vi "FPGA VI_8 Channels.vi"() -> ()   [LabVIEW 2015]
uses:
  FPGA/Injection Capture IP/Types/Injection.Timing.ctl
  FPGA/Injection Capture IP/Types/Injection.Core.Settings.ctl
  FPGA/Injection Capture IP/Types/Injection.Global.Settings.ctl
  FPGA/Injection Capture IP/Types/Injection.Mux.State.ctl
  <vilib>/Platform/TimedLoop/XDataNode/timing_clust.ctl
  <vilib>/Platform/TimedLoop/XDataNode/nitl_modes.ctl
  <vilib>/Platform/TimedLoop/XDataNode/wakeup.ctl
  FPGA/Injection Capture IP/Types/Injection.Core.Internal.Settings.ctl
  <vilib>/rvi/Emulation/niFpgaGetClockAttributes.vi
  <vilib>/rvi/Emulation/niFpgaSctlEmulationGetInTimedLoop.vi
  <vilib>/rvi/Emulation/niFpgaEmulationReportErrorSimple.vi
  <vilib>/rvi/eio/common/nirviEmuTemplateMethod_errors.vi
  <vilib>/rvi/Emulation/niFpgaCriticalErrorInLSC.vi
  <vilib>/rvi/DataTransferAndStorage/Container/Common/niFpgaContainerExecOnDevCompGetState.vi
  <vilib>/rvi/Emulation/niFpgaEmulationIsFPGAContextNoSignature.vi
  <vilib>/rvi/errors/niFpgaSetErrorForExecOnDevCompSimple.vi
  <vilib>/rvi/eio/common/nirviEmuReportErrorAndStop.vi
  <vilib>/rvi/DataTransferAndStorage/Container/Common/niFpgaContainerGetUniqueNameForEmu.vi
  <vilib>/rvi/FIFO/Fifo_Resource/nirvififoEmulationSetSize.vi
  <vilib>/rvi/FIFO/Fifo_Resource/nirviFifoEmulationQueueMgr.vi
  <instcachedir>/0/nirviFifoEmulationQueueMgr_E5CAEC123FF24DC58D834DCA3CDAA9B5.lvgen/nirviFifoEmulationQueueMgr_E5CAEC123FF24DC58D834DCA3CDAA9B5_010.vi
  <vilib>/rvi/FIFO/Fifo_Resource/nirvififoEmulationDetermineInputValidOut.vi
  <vilib>/rvi/FIFO/Fifo_Resource/nirvififoEmulationCreateLock.vi
  <vilib>/rvi/Emulation/niFpgaProcessEmulError.vi
  <vilib>/rvi/FIFO/Fifo_Resource/nirvififoEmulationObtainLock.vi
  <vilib>/rvi/FIFO/Fifo_Resource/nirvififoEmulationReleaseLock.vi
  <vilib>/rvi/occurrence/nirviWaitOnOccurrenceBase.vi
  <vilib>/rvi/errors/nirviReportUnexpectedCaseInternalError.vi
  <vilib>/rvi/errors/nirviReportUnexpectedCaseInternalError (U32).vi
  <vilib>/Utility/error.llb/Clear Errors.vi
  <vilib>/rvi/interface/RandomDataEmulation/niFpgaRandomDataHandleErrors.vi
  <instcachedir>/0/nirviFifoEmulationQueueMgr_E5CAEC123FF24DC58D834DCA3CDAA9B5.lvgen/nirviFifoEmulationQueueMgr_E5CAEC123FF24DC58D834DCA3CDAA9B5_008.vi
  <vilib>/eio/EIONode/EIONode.xnode
  <vilib>/Platform/TimedLoop/XDataNode/XDataNode.xnode
  <vilib>/rvi/DataTransferAndStorage/Container/XNode/niFpgaContainer.xnode
  <vilib>/rvi/FIFO/Fifo_Resource/niFpgaFifoEmulationRefIn.vi
  <vilib>/rvi/interface/RandomDataEmulation/nirviRandomDataFpgaReadWriteTemplate.vi
  <vilib>/Platform/TimedLoop/XDataNode/XDNodeRunTimeDep.lvlib
panel:
  in  "Settings.DMA":cluster{"# of Injectors":u8}={"# of Injectors"=6}
  out "Host DMA Out?":bool
  out "Intermediate Time Out?":bool
  in  "Settings.Index6.Injectors.Injector6":T1
  in  "Settings.Index7.Injectors.Injector7":T1
  out "Intermediate FIFO Write Timeout":bool
  in  "Settings.Global.Injectors":T2={"Enable?"=FALSE, "Initial Voltage Threshold"=12.0, "Event Dwell Limit"=2000, "Voltage Gain"=1.0, "Current Gain"=1.0, "Filter Samples"=5, "Pretrigger Samples"=5, "Active Edge"=TRUE}
  in  "Settings.Index0.Injectors.Injector0":T1
  in  "Settings.Index1.Injectors.Injector1":T1
  in  "Settings.Index2.Injectors.Injector2":T1
  in  "Settings.Index3.Injectors.Injector3":T1
  in  "Settings.Index4.Injectors.Injector4":T1
  in  "Settings.Index5.Injectors.Injector5":T1
  in  "Settings.Timing":T3={"Injection Sample Period (Ticks)"=80}
  out "Acqusition Loop Ticks":u32
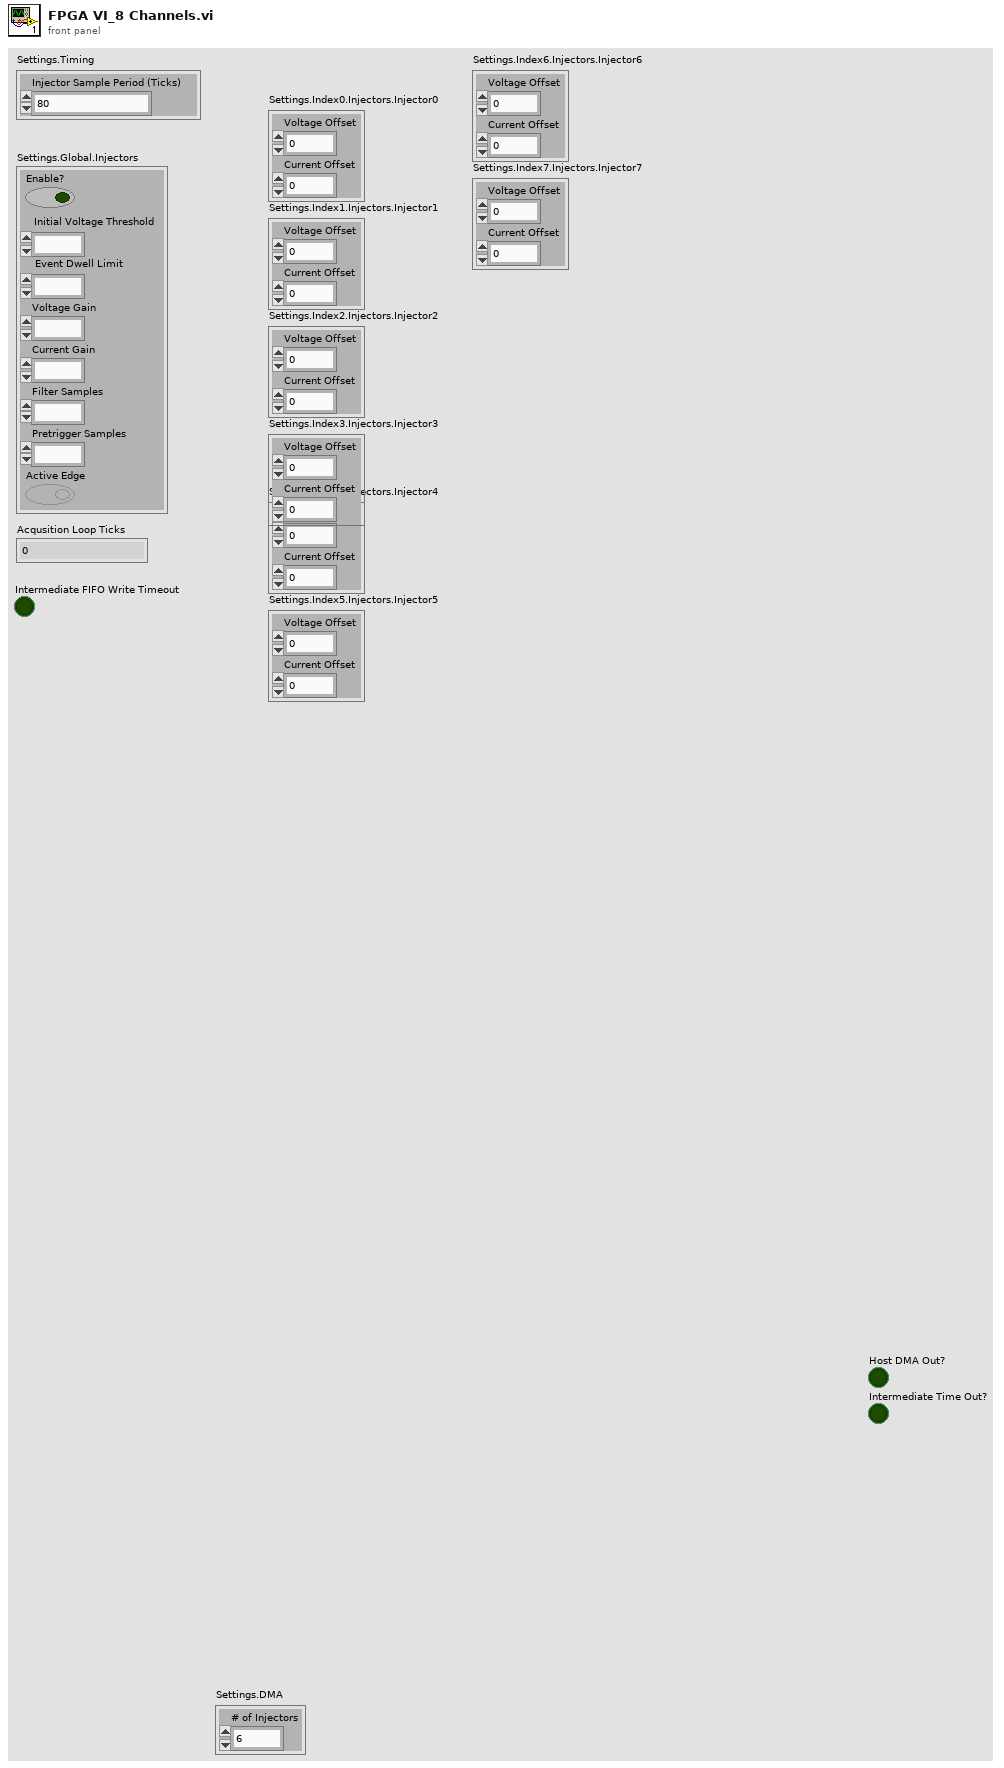
[diagram p1: front panel]
types:
  T1 = typedef "Injection.Core.Settings.ctl" = cluster{"Voltage Offset":fxp<+/-,32,8>, "Current Offset":fxp<+/-,32,8>}
  T2 = typedef "Injection.Global.Settings.ctl" = cluster{"Enable?":bool, "Initial Voltage Threshold":fxp<+/-,32,8>, "Event Dwell Limit":u16, "Voltage Gain":fxp<+/-,32,8>, "Current Gain":fxp<+/-,32,8>, "Filter Samples":u8, "Pretrigger Samples":u8, "Active Edge":bool}
  T3 = typedef "Injection.Timing.ctl" = cluster{"Injection Sample Period (Ticks)":u32}
  T4 = cluster{"Data.Samples":u32, "Injection.Period":u32, "Injector.Index":u8, "Iteration":u32}
  T5 = typedef "Injection.Mux.State.ctl" = enum8{"Wait on Transfer", "Transfer Injector Index", "Transfer # of Samples", "Transfer Injection Period", "Transfer Data Samples"}
  T6 = typedef "XDNodeRunTimeDep.lvlib/timing_clust.ctl" = cluster{"Expected End [f-1]":u64, "Actual End [f-1]":u64, "Finished Late? [f-1]":bool, "Expected End [i-1]":u64, "Actual End [i-1]":u64, "Finished Late? [i-1]":bool, "Expected Start [i]":u64, "Actual Start [i]":u64, "Expected Start [f]":u64, "Actual Start [f]":u64, "Source Name":string, "Structure Name":string, "Period":i64, "Deadline":i64, "Offset":i64, "Start":i64, "Priority":i32, "Timeout":i32, "Mode":T7, "Wakeup Reason":T8, "Error":errorcluster, "Source Type":string, "Secondary Source Type":string, "Global End Time":u64, "Global Start Time":u64, "Frame Duration":u64, "Iteration Duration":u64, "Assigned CPU":i32, "I/O Scan Engine Mode":u32}
  T7 = typedef "XDNodeRunTimeDep.lvlib/nitl_modes.ctl" = enum32{"No Change", "Process missed periods, maintain original phase", "Discard missed periods, maintain original phase", "Process missed periods, ignore original phase", "Discard missed periods, ignore original phase"}
  T8 = typedef "XDNodeRunTimeDep.lvlib/wakeup.ctl" = enum32{"Normal", "Aborted", "Asynchronous wakeup", "Timing source error", "Timed loop error", "Timeout"}
  T9 = typedef "Injection.Core.Internal.Settings.ctl" = cluster{"Data Buffer FIFO":refnum<k21>, "Capture Complete Trigger FIFO":refnum<k21>}
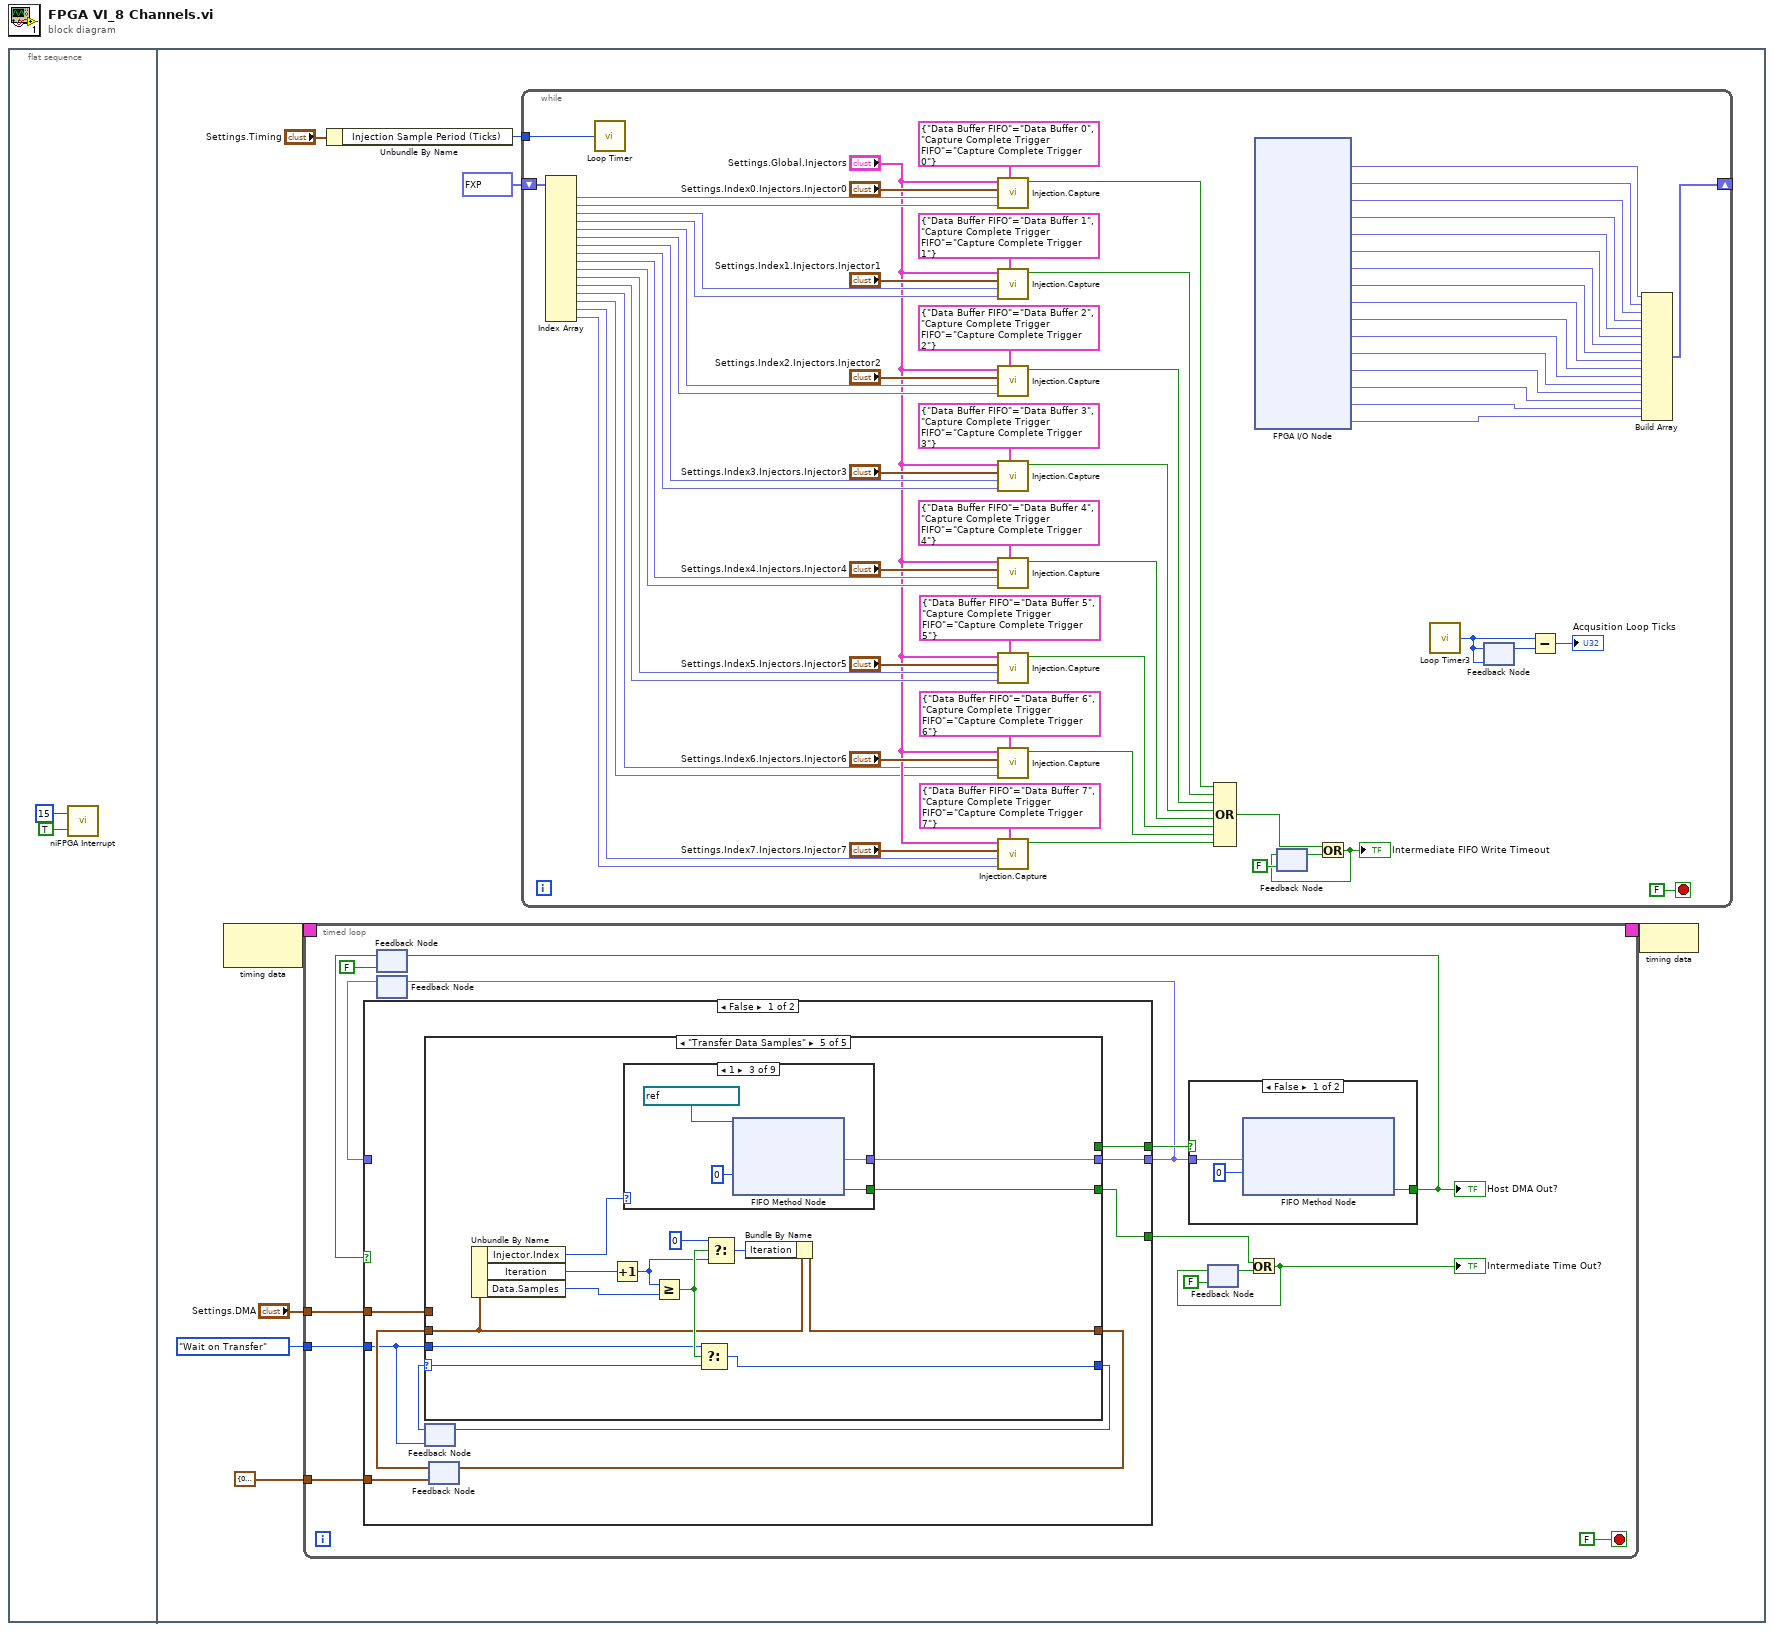
[diagram p0: block diagram]
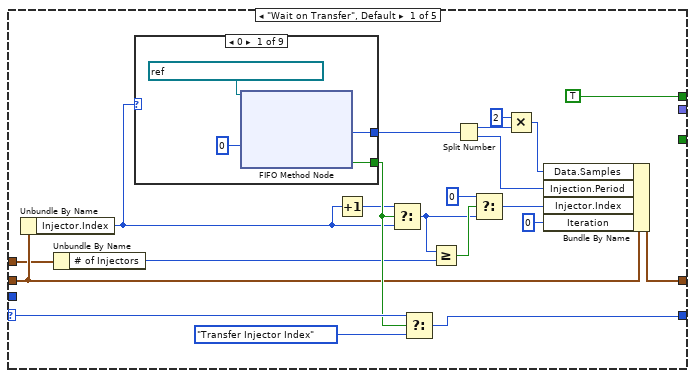
[diagram p2: hidden frame]
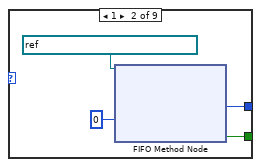
[diagram p3: hidden frame]
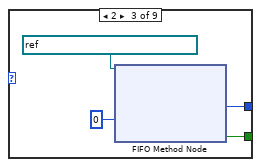
[diagram p4: hidden frame]
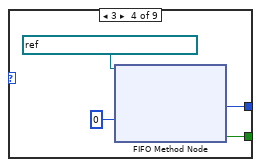
[diagram p5: hidden frame]
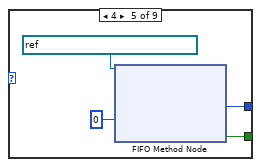
[diagram p6: hidden frame]
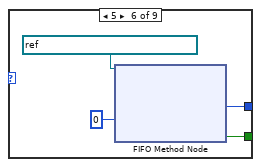
[diagram p7: hidden frame]
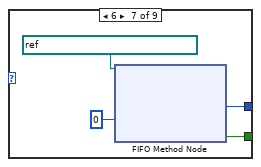
[diagram p8: hidden frame]
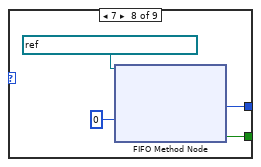
[diagram p9: hidden frame]
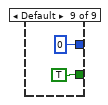
[diagram p10: hidden frame]
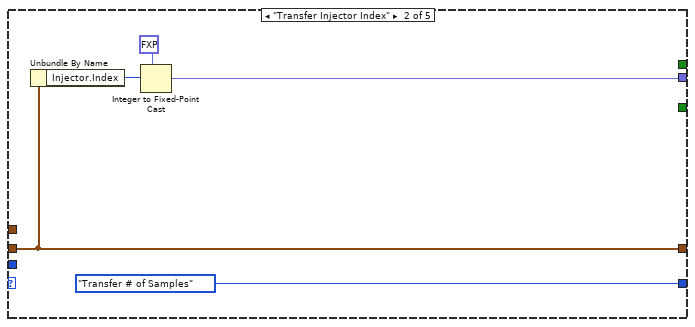
[diagram p11: hidden frame]
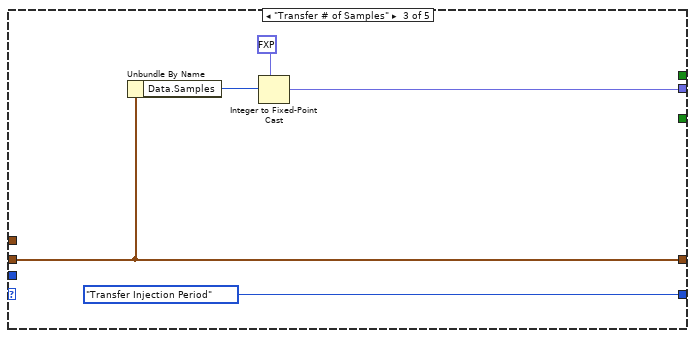
[diagram p12: hidden frame]
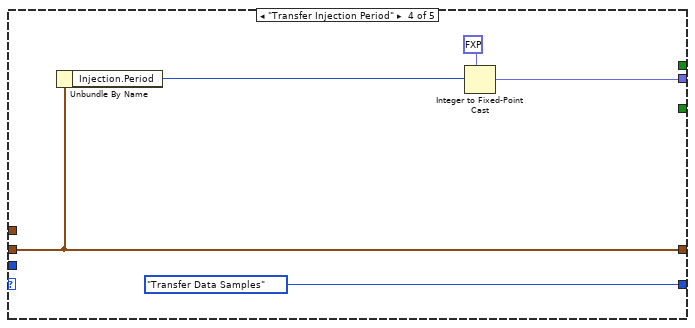
[diagram p13: hidden frame]
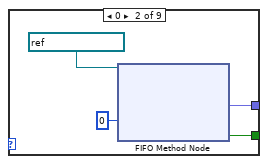
[diagram p15: hidden frame]
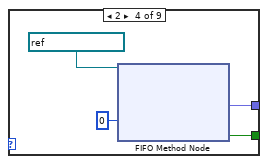
[diagram p16: hidden frame]
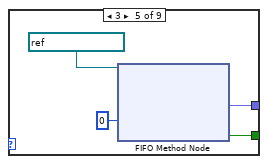
[diagram p17: hidden frame]
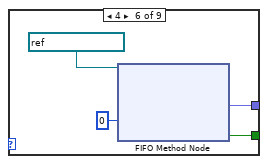
[diagram p18: hidden frame]
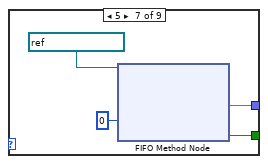
[diagram p19: hidden frame]
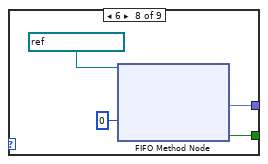
[diagram p20: hidden frame]
diagram:
  n1 = flat-sequence {
    frame #0 {
      n2 = call <vilib>:"niFPGA Interrupt.vi"("Wait Until Cleared (F)"=TRUE, "IRQ Number (0)"=u8 15) -> ()  [unwired: 1 in]
    }
    frame #1 {
      n3 = node-c288() -> (w7:T6)  [unwired: 1 in]
      n4 = timed-loop {
        timing: w7 -> [_]
        timing-out: [_] -> w6
        tunnel: "Settings.DMA" -> [w14]
        tunnel: Injection.Mux.State."Wait on Transfer" -> [w13]
        tunnel: T4 {"Data.Samples"=0, "Injection.Period"=0, "Injector.Index"=0, "Iteration"=0} ("Local.Data") -> [w12]
        stop <- FALSE stop-if-true
        n5 = feedback #1(FALSE ("Timed Out?")) -> (w22:bool)
        n6 = feedback #2() -> (w19:fxp<+/-,32,8>)  [unwired: 1 in]
        n7 = case shown="False" w22 {
          tunnel: [w34 w152] -> w20
          tunnel: [w33 w151] -> w24
          tunnel: w13 -> [w27 _]
          tunnel: [w32 w151] -> w15
          tunnel: w14 -> [w31 _]
          tunnel: w12 -> [w28 _]
          tunnel: w19 -> [_ w152]
          frame False {
            n8 = feedback #3(w27) -> (w26:T5)
            n9 = feedback #4(w28) -> (w29:T4)
            n10 = case shown="\"Transfer Data Samples\"" w26 {
              selector: w26 -> [w55 _ _ _ w112]
              tunnel: w29 -> [w46 w93 w97 w101 w110]
              tunnel: [w54 w93 w97 w101 w109] -> w30
              tunnel: [w53 Injection.Mux.State."Transfer # of Samples" Injection.Mux.State."Transfer Injection Period" Injection.Mux.State."Transfer Data Samples" w111] -> w25
              tunnel: [_ w92 w96 w103 w108] -> w34
              tunnel: [TRUE _ _ _ _] -> w33
              tunnel: w27 -> [_ _ _ _ w105]
              tunnel: [_ _ _ _ w107] -> w32
              tunnel: w31 -> [w43 _ _ _ _]
              frame "Wait on Transfer", Default {
                n11 = Unbundle By Name(w46) -> ("Injector.Index"=w45:u8)
                n12 = Unbundle By Name(w43) -> ("# of Injectors"=w42:u8)
                n13 = case shown="0" w45 {
                  tunnel: [w58 w62 w66 w70 w74 w78 w82 w86 u64 0 ("Element")] -> w41
                  tunnel: [w57 w61 w65 w69 w73 w77 w81 w85 TRUE ("Timed Out?")] -> w51
                  frame 0 {
                    n14 = xnode ("FIFO Method Node")("Timeout"=0, "FIFO In"=refnum<k21> "Capture Complete Trigger 0") -> ("Element"=w58:u64, "Timed Out?"=w57:bool)  [unwired: 1 out]
                  }
                  frame 1 {
                    n15 = xnode ("FIFO Method Node")("Timeout"=0, "FIFO In"=refnum<k21> "Capture Complete Trigger 1") -> ("Element"=w62:u64, "Timed Out?"=w61:bool)  [unwired: 1 out]
                  }
                  frame 2 {
                    n16 = xnode ("FIFO Method Node")("Timeout"=0, "FIFO In"=refnum<k21> "Capture Complete Trigger 2") -> ("Element"=w66:u64, "Timed Out?"=w65:bool)  [unwired: 1 out]
                  }
                  frame 3 {
                    n17 = xnode ("FIFO Method Node")("Timeout"=0, "FIFO In"=refnum<k21> "Capture Complete Trigger 3") -> ("Element"=w70:u64, "Timed Out?"=w69:bool)  [unwired: 1 out]
                  }
                  frame 4 {
                    n18 = xnode ("FIFO Method Node")("Timeout"=0, "FIFO In"=refnum<k21> "Capture Complete Trigger 4") -> ("Element"=w74:u64, "Timed Out?"=w73:bool)  [unwired: 1 out]
                  }
                  frame 5 {
                    n19 = xnode ("FIFO Method Node")("Timeout"=0, "FIFO In"=refnum<k21> "Capture Complete Trigger 5") -> ("Element"=w78:u64, "Timed Out?"=w77:bool)  [unwired: 1 out]
                  }
                  frame 6 {
                    n20 = xnode ("FIFO Method Node")("Timeout"=0, "FIFO In"=refnum<k21> "Capture Complete Trigger 6") -> ("Element"=w82:u64, "Timed Out?"=w81:bool)  [unwired: 1 out]
                  }
                  frame 7 {
                    n21 = xnode ("FIFO Method Node")("Timeout"=0, "FIFO In"=refnum<k21> "Capture Complete Trigger 7") -> ("Element"=w86:u64, "Timed Out?"=w85:bool)  [unwired: 1 out]
                  }
                  frame Default {
                  }
                }
                n22 = Increment(x=w45) -> (x+1=w50:u8)
                n23 = Select(t=w50, s=w51, f=w45) -> (s? t:f=w48:u8)
                n24 = Select(t=w55, s=w51, f=Injection.Mux.State."Transfer Injector Index") -> (s? t:f=w53:T5)
                n25 = Greater Or Equal?(x=w48, y=w42) -> (x >= y?=w49:bool)
                n26 = Split Number(x=w41) -> (hi(x)=w40:u32, lo(x)=w39:u32)
                n27 = Select(t=u8 0, s=w49, f=w48) -> (s? t:f=w44:u8)
                n28 = Multiply(x=u32 2, y=w40) -> (x*y=w37:u32)
                n29 = Bundle By Name(cluster=w46, "Data.Samples"=w37, "Injection.Period"=w39, "Injector.Index"=w44, "Iteration"=u32 0) -> (w54:T4)
              }
              frame "Transfer Injector Index" {
                n30 = Unbundle By Name(w93) -> ("Injector.Index"=w94:u8)
                n31 = Integer to Fixed-Point Cast(fixed-point type=fxp<+/-,32,8> 0.0, integer=w94) -> (fixed-point=w92:fxp<+/-,32,8>)
              }
              frame "Transfer # of Samples" {
                n32 = Unbundle By Name(w97) -> ("Data.Samples"=w98:u32)
                n33 = Integer to Fixed-Point Cast(fixed-point type=fxp<+/-,32,8> 0.0, integer=w98) -> (fixed-point=w96:fxp<+/-,32,8>)
              }
              frame "Transfer Injection Period" {
                n34 = Unbundle By Name(w101) -> ("Injection.Period"=w102:u32)
                n35 = Integer to Fixed-Point Cast(fixed-point type=fxp<+/-,32,8> 0.0, integer=w102) -> (fixed-point=w103:fxp<+/-,32,8>)
              }
              frame "Transfer Data Samples" {
                n36 = Unbundle By Name(w110) -> ("Injector.Index"=w118:u8, "Iteration"=w113:u32, "Data.Samples"=w106:u32)
                n37 = Increment(x=w113) -> (x+1=w115:u32)
                n38 = case shown="1" w118 {
                  tunnel: [_ w121 w125 w129 w133 w137 w141 w145 w149] -> w108
                  tunnel: [_ w120 w124 w128 w132 w136 w140 w144 w148] -> w107
                  frame Default {
                  }
                  frame 0 {
                    n39 = xnode ("FIFO Method Node")("Timeout"=0, "FIFO In"=refnum<k21> "Data Buffer 0" ("Voltage FIFO")) -> ("Element"=w121:fxp<+/-,32,8>, "Timed Out?"=w120:bool)  [unwired: 1 out]
                  }
                  frame 1 {
                    n40 = xnode ("FIFO Method Node")("Timeout"=0, "FIFO In"=refnum<k21> "Data Buffer 1" ("Voltage FIFO")) -> ("Element"=w125:fxp<+/-,32,8>, "Timed Out?"=w124:bool)  [unwired: 1 out]
                  }
                  frame 2 {
                    n41 = xnode ("FIFO Method Node")("Timeout"=0, "FIFO In"=refnum<k21> "Data Buffer 2" ("Voltage FIFO")) -> ("Element"=w129:fxp<+/-,32,8>, "Timed Out?"=w128:bool)  [unwired: 1 out]
                  }
                  frame 3 {
                    n42 = xnode ("FIFO Method Node")("Timeout"=0, "FIFO In"=refnum<k21> "Data Buffer 3" ("Voltage FIFO")) -> ("Element"=w133:fxp<+/-,32,8>, "Timed Out?"=w132:bool)  [unwired: 1 out]
                  }
                  frame 4 {
                    n43 = xnode ("FIFO Method Node")("Timeout"=0, "FIFO In"=refnum<k21> "Data Buffer 4" ("Voltage FIFO")) -> ("Element"=w137:fxp<+/-,32,8>, "Timed Out?"=w136:bool)  [unwired: 1 out]
                  }
                  frame 5 {
                    n44 = xnode ("FIFO Method Node")("Timeout"=0, "FIFO In"=refnum<k21> "Data Buffer 5" ("Voltage FIFO")) -> ("Element"=w141:fxp<+/-,32,8>, "Timed Out?"=w140:bool)  [unwired: 1 out]
                  }
                  frame 6 {
                    n45 = xnode ("FIFO Method Node")("Timeout"=0, "FIFO In"=refnum<k21> "Data Buffer 6" ("Voltage FIFO")) -> ("Element"=w145:fxp<+/-,32,8>, "Timed Out?"=w144:bool)  [unwired: 1 out]
                  }
                  frame 7 {
                    n46 = xnode ("FIFO Method Node")("Timeout"=0, "FIFO In"=refnum<k21> "Data Buffer 7" ("Voltage FIFO")) -> ("Element"=w149:fxp<+/-,32,8>, "Timed Out?"=w148:bool)  [unwired: 1 out]
                  }
                }
                n47 = Greater Or Equal?(x=w115, y=w106) -> (x >= y?=w117:bool)
                n48 = Select(t=w105, s=w117, f=w112) -> (s? t:f=w111:T5)
                n49 = Select(t=u32 0, s=w117, f=w115) -> (s? t:f=w114:u32)
                n50 = Bundle By Name(cluster=w110, "Iteration"=w114) -> (w109:T4)
              }
            }
            n51 = feedback-in #3(w25) -> ()
            n52 = feedback-in #4(w30) -> ()
          }
          frame True {
            w151 = FALSE
          }
        }
        n53 = feedback-in #2(w20) -> ()
        n54 = case shown="False" w24 {
          tunnel: w20 -> [w154 _]
          tunnel: [w153 FALSE ("Timed Out?")] -> w23
          frame False {
            n55 = xnode ("FIFO Method Node")("Element"=w154, "Timeout"=0) -> ("Timed Out?"=w153:bool)  [unwired: 1 in, 1 out]
          }
          frame True {
          }
        }
        "Host DMA Out?" <- w23
        n56 = feedback-in #1(w23) -> ()
        n57 = feedback #5(FALSE ("Timed Out?")) -> (w17:bool)
        n58 = Or(x=w15, y=w17) -> (x .or. y?=w16:bool)
        "Intermediate Time Out?" <- w16
        n59 = feedback-in #5(w16) -> ()
      }
      n60 = Unbundle By Name("Settings.Timing") -> ("Injection Sample Period (Ticks)"=w8:u32)
      n61 = while {
        shift-right: [w189] -> _
        shift-left: fxp<+/-,24,5>[] [0.0, 0.0, 0.0, 0.0, 0.0, 0.0, 0.0, 0.0, 0.0, 0.0, 0.0, 0.0, 0.0, 0.0, 0.0, 0.0] -> [w209]
        tunnel: w8 -> [w177]
        stop <- FALSE stop-if-true
        n62 = Index Array(array=w209) -> (element #1=w220:fxp<+/-,24,5>, element #2=w221:fxp<+/-,24,5>, element #3=w218:fxp<+/-,24,5>, element #4=w219:fxp<+/-,24,5>, element #5=w216:fxp<+/-,24,5>, element #6=w217:fxp<+/-,24,5>, element #7=w214:fxp<+/-,24,5>, element #8=w215:fxp<+/-,24,5>, element #9=w212:fxp<+/-,24,5>, element #10=w213:fxp<+/-,24,5>, element #11=w210:fxp<+/-,24,5>, element #12=w211:fxp<+/-,24,5>, element #13=w181:fxp<+/-,24,5>, element #14=w180:fxp<+/-,24,5>, element #15=w179:fxp<+/-,24,5>, element #16=w178:fxp<+/-,24,5>)  [unwired: 16 in]
        n63 = call "Loop Timer"("Count(Ticks)"=w177) -> ()  [unwired: 1 out]
        n64 = call "Injection.Capture.vi"("FIFOs"=T9 {"Data Buffer FIFO"="Data Buffer 0", "Capture Complete Trigger FIFO"="Capture Complete Trigger 0"} ("InjectorCore.Settings"), "Current (PreScaled)"=w221, "Voltage (PreScaled)"=w220, "Settings.Index<#>.<Group>.<UserName>"="Settings.Index0.Injectors.Injector0", "Settings.Global.<Group>"="Settings.Global.Injectors") -> ("Intermediate FIFO Timeout?"=w228:bool)  [unwired: 4 in, 2 out]
        n65 = call "Injection.Capture.vi"("FIFOs"=T9 {"Data Buffer FIFO"="Data Buffer 1", "Capture Complete Trigger FIFO"="Capture Complete Trigger 1"} ("InjectorCore.Settings"), "Current (PreScaled)"=w219, "Voltage (PreScaled)"=w218, "Settings.Index<#>.<Group>.<UserName>"="Settings.Index1.Injectors.Injector1", "Settings.Global.<Group>"="Settings.Global.Injectors") -> ("Intermediate FIFO Timeout?"=w227:bool)  [unwired: 4 in, 2 out]
        n66 = call "Injection.Capture.vi"("FIFOs"=T9 {"Data Buffer FIFO"="Data Buffer 2", "Capture Complete Trigger FIFO"="Capture Complete Trigger 2"} ("InjectorCore.Settings"), "Current (PreScaled)"=w217, "Voltage (PreScaled)"=w216, "Settings.Index<#>.<Group>.<UserName>"="Settings.Index2.Injectors.Injector2", "Settings.Global.<Group>"="Settings.Global.Injectors") -> ("Intermediate FIFO Timeout?"=w226:bool)  [unwired: 4 in, 2 out]
        n67 = call "Injection.Capture.vi"("FIFOs"=T9 {"Data Buffer FIFO"="Data Buffer 3", "Capture Complete Trigger FIFO"="Capture Complete Trigger 3"} ("InjectorCore.Settings"), "Current (PreScaled)"=w215, "Voltage (PreScaled)"=w214, "Settings.Index<#>.<Group>.<UserName>"="Settings.Index3.Injectors.Injector3", "Settings.Global.<Group>"="Settings.Global.Injectors") -> ("Intermediate FIFO Timeout?"=w225:bool)  [unwired: 4 in, 2 out]
        n68 = call "Injection.Capture.vi"("FIFOs"=T9 {"Data Buffer FIFO"="Data Buffer 4", "Capture Complete Trigger FIFO"="Capture Complete Trigger 4"} ("InjectorCore.Settings"), "Current (PreScaled)"=w213, "Voltage (PreScaled)"=w212, "Settings.Index<#>.<Group>.<UserName>"="Settings.Index4.Injectors.Injector4", "Settings.Global.<Group>"="Settings.Global.Injectors") -> ("Intermediate FIFO Timeout?"=w224:bool)  [unwired: 4 in, 2 out]
        n69 = call "Injection.Capture.vi"("FIFOs"=T9 {"Data Buffer FIFO"="Data Buffer 5", "Capture Complete Trigger FIFO"="Capture Complete Trigger 5"} ("InjectorCore.Settings"), "Current (PreScaled)"=w211, "Voltage (PreScaled)"=w210, "Settings.Index<#>.<Group>.<UserName>"="Settings.Index5.Injectors.Injector5", "Settings.Global.<Group>"="Settings.Global.Injectors") -> ("Intermediate FIFO Timeout?"=w223:bool)  [unwired: 4 in, 2 out]
        n70 = call "Injection.Capture.vi"("FIFOs"=T9 {"Data Buffer FIFO"="Data Buffer 6", "Capture Complete Trigger FIFO"="Capture Complete Trigger 6"} ("InjectorCore.Settings"), "Current (PreScaled)"=w180, "Voltage (PreScaled)"=w181, "Settings.Index<#>.<Group>.<UserName>"="Settings.Index6.Injectors.Injector6", "Settings.Global.<Group>"="Settings.Global.Injectors") -> ("Intermediate FIFO Timeout?"=w183:bool)  [unwired: 4 in, 2 out]
        n71 = call "Injection.Capture.vi"("FIFOs"=T9 {"Data Buffer FIFO"="Data Buffer 7", "Capture Complete Trigger FIFO"="Capture Complete Trigger 7"} ("InjectorCore.Settings"), "Current (PreScaled)"=w178, "Voltage (PreScaled)"=w179, "Settings.Index<#>.<Group>.<UserName>"="Settings.Index7.Injectors.Injector7", "Settings.Global.<Group>"="Settings.Global.Injectors") -> ("Intermediate FIFO Timeout?"=w182:bool)  [unwired: 4 in, 2 out]
        n72 = Compound Arithmetic op=OR(w228, w227, w226, w225, w224, w223, w183, w182) -> (w199:bool)
        n73 = xnode "FPGA I/O Node"() -> ("Mod1/AI0"=w176:fxp<+/-,24,5>, "Mod1/AI1"=w175:fxp<+/-,24,5>, "Mod1/AI2"=w174:fxp<+/-,24,5>, "Mod1/AI3"=w173:fxp<+/-,24,5>, "Mod2/AI0"=w172:fxp<+/-,24,5>, "Mod2/AI1"=w171:fxp<+/-,24,5>, "Mod2/AI2"=w170:fxp<+/-,24,5>, "Mod2/AI3"=w169:fxp<+/-,24,5>, "Mod3/AI0"=w168:fxp<+/-,24,5>, "Mod3/AI1"=w167:fxp<+/-,24,5>, "Mod3/AI2"=w166:fxp<+/-,24,5>, "Mod3/AI3"=w165:fxp<+/-,24,5>, "Mod4/AI0"=w164:fxp<+/-,24,5>, "Mod4/AI1"=w163:fxp<+/-,24,5>, "Mod4/AI2"=w162:fxp<+/-,24,5>, "Mod4/AI3"=w161:fxp<+/-,24,5>)  [unwired: 16 in, 16 out]
        n74 = feedback #6(FALSE ("Timed Out?")) -> (w200:bool)
        n75 = Or(x=w199, y=w200) -> (x .or. y?=w198:bool)
        "Intermediate FIFO Write Timeout" <- w198
        n76 = feedback-in #6(w198) -> ()
        n77 = call "Loop Timer3"() -> ("Tick Count(Ticks)"=w195:u32)  [unwired: 1 in]
        n78 = feedback #7(w195) -> (w197:u32)
        n79 = feedback-in #7(w195) -> ()
        n80 = Subtract(x=w195, y=w197) -> (x-y=→"Acqusition Loop Ticks":u32)
        n81 = Build Array(w176, w175, w174, w173, w172, w171, w170, w169, w168, w167, w166, w165, w164, w163, w162, w161) -> (w189:fxp<+/-,24,5>[])
      }
      n82 = node-c288(w6) -> ()
    }
  }
